vi "PWM_Waveform_Analysis_v1.vi"(6 "Waveform":waveform(dbl)[](array[waveform]), 8 "Duty Cycle":i32=25, 9 "Active Leg":i32, 10 "Analysis Leg":i32) -> (2 "Message":string, 3 "Result (Boolean)":bool)   [LabVIEW 2019]
uses:
  <vilib>/measure/NI_MAPro.lvlib
  <vilib>/measure/mascope.llb/Pulse Measurements 1 chan.vi
  <vilib>/measure/madcrms.llb/Basic Averaged DC-RMS for 1 Chan.vi
  Ctls/Controlboard_Select.ctl
panel:
  in  "Board Selector":T1
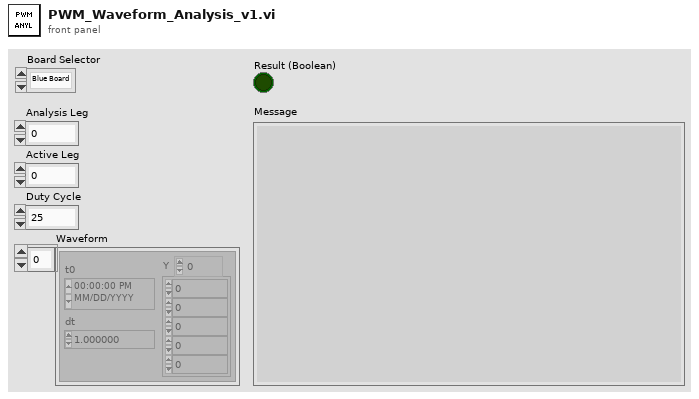
[diagram p1: front panel]
types:
  T1 = typedef "Controlboard_Select.ctl" = enum16{"Blue Board", "Green Board"}
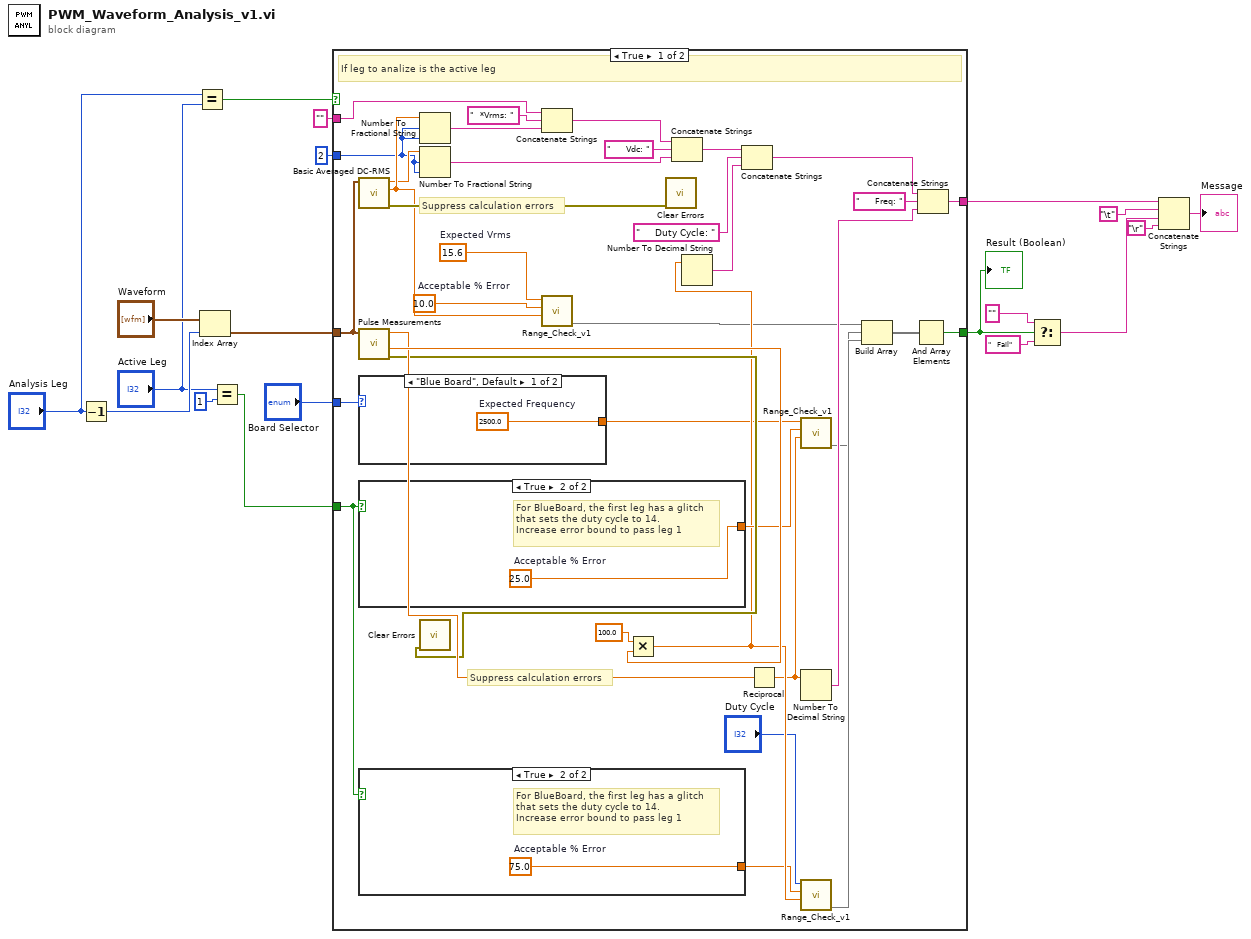
[diagram p0: block diagram]
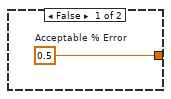
[diagram p2: hidden frame]
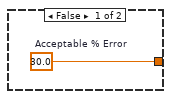
[diagram p3: hidden frame]
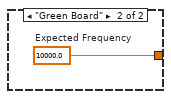
[diagram p4: hidden frame]
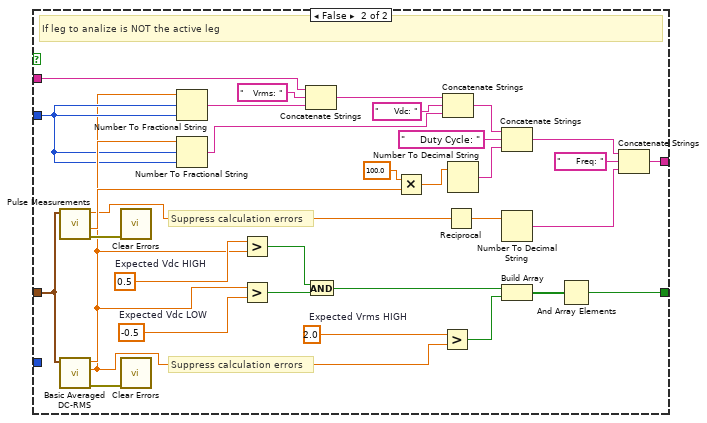
[diagram p5: hidden frame]
diagram:
  n1 = Decrement(x="Analysis Leg") -> (x-1=w19:i32)
  n2 = Equal?(x="Analysis Leg", y="Active Leg") -> (x = y?=w9:bool)
  n3 = Index Array(array="Waveform", index=w19) -> (element=w14:waveform(dbl))
  n4 = Equal?(x="Active Leg", y=1) -> (x = y?=w2:bool)
  n5 = case shown="True" w9 {
    tunnel: w14 -> [w41 w83]
    tunnel: [w35 w80] -> w3
    tunnel: [w24 w67] -> w10
    tunnel: "" -> [w26 w69]
    tunnel: 2 -> [w23 w66]
    tunnel: w2 -> [w21 _]
    tunnel: "Board Selector" -> [w20 _]
    frame True {
      w29 = 10.0  # Acceptable % Error
      w28 = 15.6  # Expected Vrms
      # "Suppress calculation errors"
      # "Suppress calculation errors"
      # "If leg to analize is the active leg"
      n6 = call-poly <vilib>:"Basic Averaged DC-RMS.vi"("signal in"=w41) -> ("error out"=w42:errorcluster, "RMS value"=w37:dbl, "DC value"=w27:dbl)  [unwired: 7 in, 1 out]
      n7 = call-poly <vilib>:"Pulse Measurements.vi"("signal in"=w41) -> ("error out"=w51:errorcluster, "duty cycle"=w53:dbl, "period"=w52:dbl)  [unwired: 6 in, 2 out]
      n8 = case shown="\"Blue Board\", Default" w20 {
        tunnel: [w61 w62] -> w46
        frame "Blue Board", Default {
          w61 = 2500.0  # Expected Frequency
        }
        frame "Green Board" {
          w62 = 10000.0  # Expected Frequency
        }
      }
      n9 = case shown="True" w21 {
        tunnel: [w57 w58] -> w50
        frame False {
          w57 = 0.5  # Acceptable % Error
        }
        frame True {
          w58 = 25.0  # Acceptable % Error
          # "For BlueBoard, the first leg has a glitch\nthat sets the duty cycle to 14.\nIncrease error bound to pass leg 1"
        }
      }
      n10 = case shown="True" w21 {
        tunnel: [w59 w60] -> w22
        frame False {
          w59 = 30.0  # Acceptable % Error
        }
        frame True {
          w60 = 75.0  # Acceptable % Error
          # "For BlueBoard, the first leg has a glitch\nthat sets the duty cycle to 14.\nIncrease error bound to pass leg 1"
        }
      }
      n11 = Number To Fractional String(number=w37, width (-)=w23, precision (6)=w23) -> (F-format string=w39:string)  [unwired: 1 in]
      n12 = Number To Fractional String(number=w27, width (-)=w23, precision (6)=w23) -> (F-format string=w33:string)  [unwired: 1 in]
      n13 = call <vilib>:"Clear Errors.vi"("error in (no error)"=w51) -> ()  [unwired: 5 in, 2 out]
      n14 = Concatenate Strings(w26, "  *Vrms: " ("string"), w39) -> (w31:string)
      n15 = call "Range_Check_v1.vi"("Actual Value"=w37, "Acceptable% Error"=w29, "Expected Value"=w28) -> (0:w40)  [unwired: 6 in, 2 out]
      n16 = Multiply(x=100.0, y=w53) -> (x*y=w47:dbl)
      n17 = call <vilib>:"Clear Errors.vi"("error in (no error)"=w42) -> ()  [unwired: 5 in, 2 out]
      n18 = Concatenate Strings(w31, "     Vdc: " ("string"), w33) -> (w25:string)
      n19 = Number To Decimal String(number=w47) -> (decimal integer string=w48:string)  [unwired: 1 in]
      n20 = Concatenate Strings(w25, "     Duty Cycle: " ("string"), w48) -> (w32:string)
      n21 = Reciprocal(x=w52) -> (1/x=w43:dbl)
      n22 = call "Range_Check_v1.vi"("Actual Value"=w43, "Acceptable% Error"=w50, "Expected Value"=w46) -> (0:w36)  [unwired: 6 in, 2 out]
      n23 = Number To Decimal String(number=w43) -> (decimal integer string=w44:string)  [unwired: 1 in]
      n24 = call "Range_Check_v1.vi"("Actual Value"=w47, "Acceptable% Error"=w22, "Expected Value"="Duty Cycle") -> (0:w54)  [unwired: 6 in, 2 out]
      n25 = Build Array(w40, w36, w54) -> (w55:void[])
      n26 = And Array Elements(Boolean array=w55) -> (logical AND=w35:bool)
      n27 = Concatenate Strings(w32, "     Freq: " ("string"), w44) -> (w24:string)
    }
    frame False {
      w65 = 2.0  # Expected Vrms HIGH
      w74 = -0.5  # Expected Vdc LOW
      w75 = 0.5  # Expected Vdc HIGH
      # "Suppress calculation errors"
      # "Suppress calculation errors"
      # "If leg to analize is NOT the active leg"
      n28 = call-poly <vilib>:"Pulse Measurements.vi"("signal in"=w83) -> ("error out"=w91:errorcluster, "duty cycle"=w93:dbl, "period"=w92:dbl)  [unwired: 6 in, 2 out]
      n29 = call-poly <vilib>:"Basic Averaged DC-RMS.vi"("signal in"=w83) -> ("error out"=w84:errorcluster, "RMS value"=w64:dbl, "DC value"=w70:dbl)  [unwired: 7 in, 1 out]
      n30 = call <vilib>:"Clear Errors.vi"("error in (no error)"=w91) -> ()  [unwired: 5 in, 2 out]
      n31 = call <vilib>:"Clear Errors.vi"("error in (no error)"=w84) -> ()  [unwired: 5 in, 2 out]
      n32 = Number To Fractional String(number=w64, width (-)=w66, precision (6)=w66) -> (F-format string=w82:string)  [unwired: 1 in]
      n33 = Number To Fractional String(number=w70, width (-)=w66, precision (6)=w66) -> (F-format string=w78:string)  [unwired: 1 in]
      n34 = Greater?(x=w75, y=w70) -> (0:w73:bool)
      n35 = Greater?(x=w70, y=w74) -> (0:w72:bool)
      n36 = Concatenate Strings(w69, "   Vrms: " ("string"), w82) -> (w76:string)
      n37 = And(x=w73, y=w72) -> (x .and. y?=w71:bool)
      n38 = Multiply(x=100.0, y=w93) -> (x*y=w88:dbl)
      n39 = Greater?(x=w65, y=w64) -> (0:w63:bool)
      n40 = Concatenate Strings(w76, "     Vdc: " ("string"), w78) -> (w68:string)
      n41 = Reciprocal(x=w92) -> (1/x=w85:dbl)
      n42 = Number To Decimal String(number=w88) -> (decimal integer string=w89:string)  [unwired: 1 in]
      n43 = Concatenate Strings(w68, "     Duty Cycle: " ("string"), w89) -> (w77:string)
      n44 = Number To Decimal String(number=w85) -> (decimal integer string=w86:string)  [unwired: 1 in]
      n45 = Build Array(w71, w63) -> (w94:bool[])
      n46 = And Array Elements(Boolean array=w94) -> (logical AND=w80:bool)
      n47 = Concatenate Strings(w77, "     Freq: " ("string"), w86) -> (w67:string)
    }
  }
  "Result (Boolean)" <- w3
  n48 = Select(t="" ("string"), s=w3, f="   Fail" ("string")) -> (s? t:f=w11:string)
  n49 = Concatenate Strings(w10, "\t", w11, "\r") -> (→"Message":string)
